vi "Set Dump Switch.vi"(4 "error in":errorcluster, 6 "Earth":bool) -> (0 "error out":errorcluster)   [LabVIEW 2015]
uses:
  <vilib>/DAQmx/write.llb/DAQmx Write (Digital Bool 1Line 1Point).vi
  <vilib>/DAQmx/miscellaneous.llb/DAQmx Fill In Error Info.vi
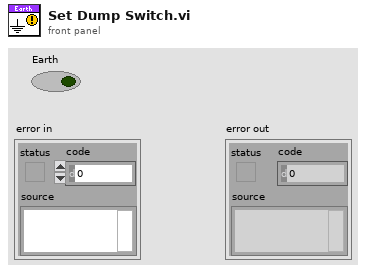
[diagram p1: front panel]
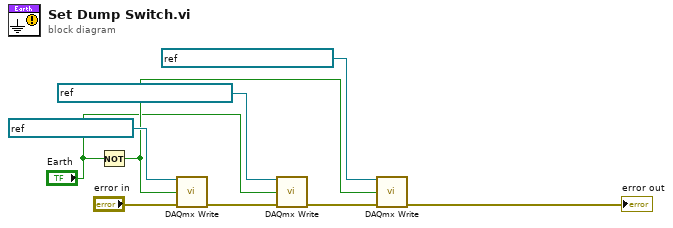
[diagram p0: block diagram]
diagram:
  n1 = Not(x="Earth") -> (.not. x?=w3:bool)
  n2 = call-poly <vilib>:"DAQmx Write.vi"("task/channels in"=refnum<k21> "DO4 Dump Switch" ("DAQmx Global Channel"), "data"=w3, "error in"="error in") -> ("error out"=w6:errorcluster)  [unwired: 10 in, 2 out]
  n3 = call-poly <vilib>:"DAQmx Write.vi"("task/channels in"=refnum<k21> "DO6 Enclosure Earthed light" ("DAQmx Global Channel"), "data"="Earth", "error in"=w6) -> ("error out"=w5:errorcluster)  [unwired: 10 in, 2 out]
  n4 = call-poly <vilib>:"DAQmx Write.vi"("task/channels in"=refnum<k21> "DO5 Enclosure HV ON light" ("DAQmx Global Channel"), "data"=w3, "error in"=w5) -> ("error out"=→"error out":errorcluster)  [unwired: 10 in, 2 out]
